vi "IIC Slave Read Bytes.vi"(9 "TimeOutMs":i32, 10 "IICIndex":i32, 11 "DevIndex":i32) -> (2 "function return":i32, 3 "pReadData":u8[](array[numeric]))   [LabVIEW 2010, in "usb2iic.lvlib"]
doc: "int WINAPI IIC_SlaveReadBytes(int DevIndex,int IICIndex,unsigned char *pReadData,int TimeOutMs);"
uses:
  usb2iic.lvlib
  USB2XXX.dll
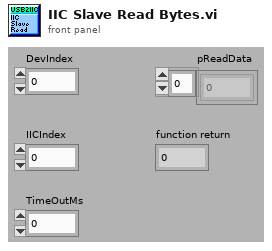
[diagram p1: front panel]
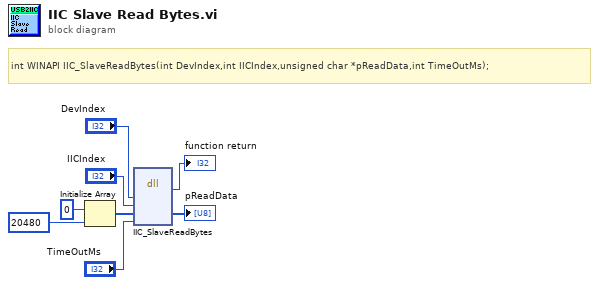
[diagram p0: block diagram]
diagram:
  # "int WINAPI IIC_SlaveReadBytes(int DevIndex,int IICIndex,unsigned char *pReadData,int TimeOutMs);"
  n1 = Initialize Array(u8 0 ("element"), 20480 ("dimension size")) -> (w5:u8[])
  n2 = dll-call lib="G:/OtherWork/USB2XXX_Example/trunk/Labview/PublicFiles/usb2iic/USB2XXX.*" fn="IIC_SlaveReadBytes"("DevIndex"="DevIndex", "IICIndex"="IICIndex", "pReadData"=w5, "TimeOutMs"="TimeOutMs") -> (→"function return":i32, "pReadData"=→"pReadData":u8[])  [unwired: 6 in, 2 out]
